vi "数值比较.vi"() -> ()   [LabVIEW 2022 SP3]
doc: "本VI是为《我和LabVIEW》一书编写的示例。\n关于本书的介绍请参考网页：\nhttp://ruanqizhen.spaces.live.com/blog/cns!5852D4F797C53FB6!4310.entry"
panel:
  in  "b":i32
  in  "a":i32
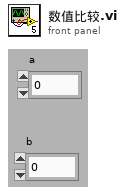
[diagram p1: front panel]
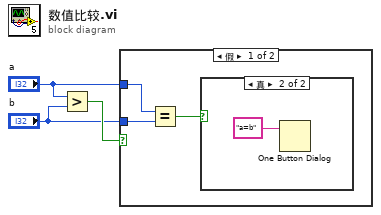
[diagram p0: block diagram]
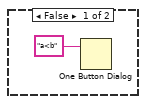
[diagram p2: hidden frame]
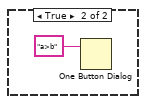
[diagram p3: hidden frame]
diagram:
  n1 = Greater?(x="a", y="b") -> (0:w3:bool)
  n2 = case shown="假" w3 {
    tunnel: "a" -> [w6 _]
    tunnel: "b" -> [w5 _]
    frame False {
      n3 = Equal?(x=w6, y=w5) -> (x = y?=w4:bool)
      n4 = case shown="真" w4 {
        frame False {
          n5 = One Button Dialog(message="a<b") -> ()  [unwired: 2 out]
        }
        frame True {
          n6 = One Button Dialog(message="a=b") -> ()  [unwired: 2 out]
        }
      }
    }
    frame True {
      n7 = One Button Dialog(message="a>b") -> ()  [unwired: 2 out]
    }
  }
